vi "hysteresis.vi"(1 "Size":i16, 2 "In":i16) -> (0 "Out":i16)   [LabVIEW 2010, in "Wall Follower.lvrbt"]
uses:
  Wall Follower.lvrbt
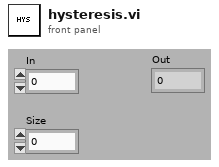
[diagram p1: front panel]
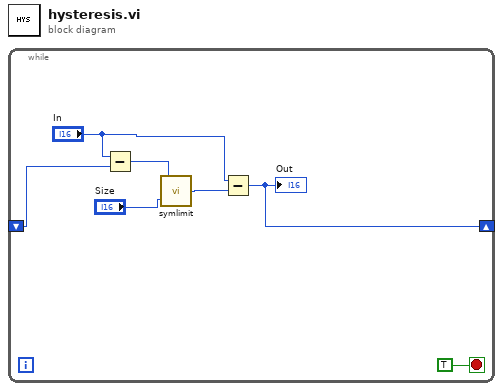
[diagram p0: block diagram]
diagram:
  n1 = while {
    shift-right: [w4] -> _
    shift-left: _ -> [w1]
    stop <- TRUE stop-if-true
    n2 = Subtract(x="In", y=w1) -> (x-y=w2:i16)
    n3 = call "symlimit.vi"("Limit"="Size", "Input Sig"=w2) -> ("Output Sig"=w5:i16)
    n4 = Subtract(x="In", y=w5) -> (x-y=w4:i16)
    "Out" <- w4
  }
